vi "deploy alarm map.vi"() -> ()   [LabVIEW 2016, in "opSignIn.lvlib"]
uses:
  opSignIn.lvlib
  alarmMap.ctl
panel:
  in  "导入":bool
  in  "导出":bool
  in  "Project":i32(listbox)
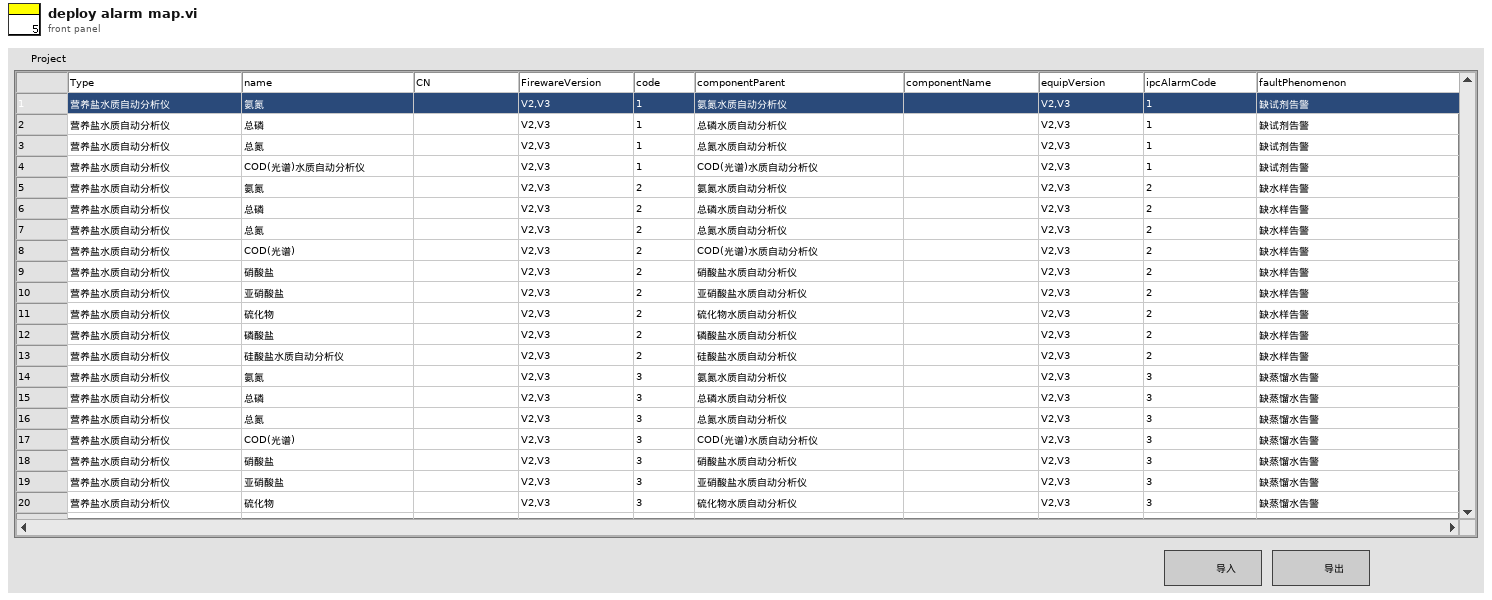
[diagram p1: front panel]
types:
  T1 = typedef "opSignIn.lvlib/alarmMap.ctl" = cluster{"name":string, "componentParentPath":string, "componentName":string, "equipVersion":string, "ipcAlarmCode":string, "faultName":string, "是否上报":string}
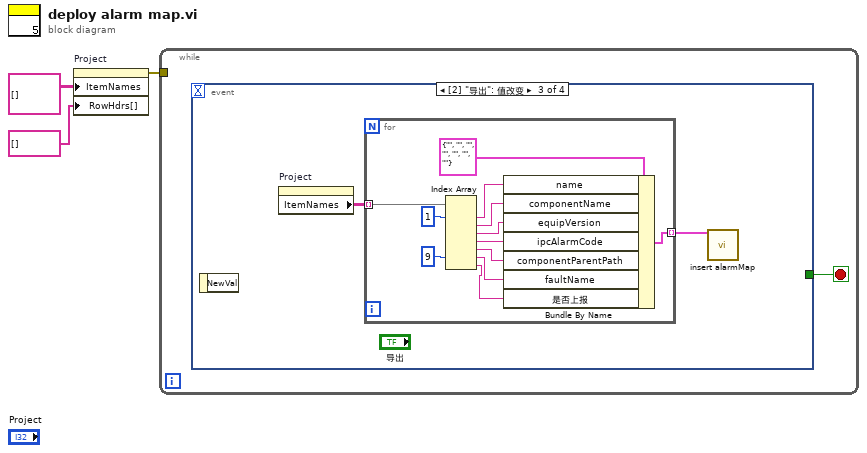
[diagram p0: block diagram]
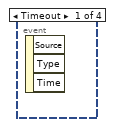
[diagram p2: hidden frame]
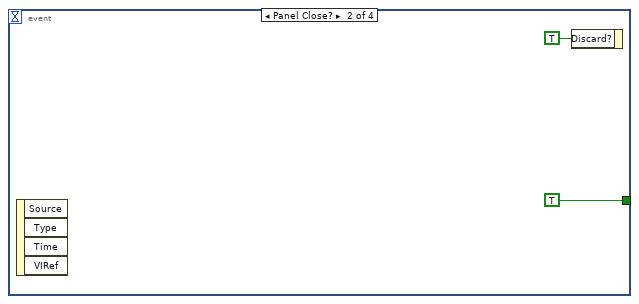
[diagram p3: hidden frame]
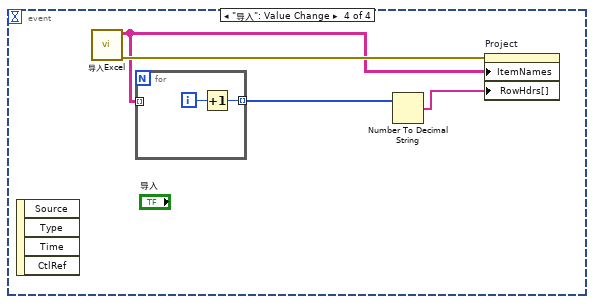
[diagram p4: hidden frame]
diagram:
  n1 = property on="Project" class="MCListbox (严格)"("ItemNames"=string[][] [] ("项名"), "RowHdrs[]"=string[] [] ("行首字符串[]")) -> (error out=w1:errorcluster)  [unwired: 2 in, 1 out]
  n2 = while {
    tunnel: w1 -> [_]
    stop <- w4 stop-if-true
    n3 = event shown="[2] \"导出\": 值改变" {
      selector: _ -> [_ _ _ _]
      dyn-events: _ -> [_ _ _ _]
      timeout: _ -> [_ _ _ _]
      tunnel: [_ TRUE _ _] -> w4
      event Timeout {
        n4 = event-data() -> ()  [unwired: 1 in, 3 out]
      }
      event Panel Close? {
        n5 = event-data() -> ()  [unwired: 1 in, 4 out]
        n6 = event-data("Discard?"=TRUE ("放弃？")) -> ()  [unwired: 1 in, 1 out]
      }
      event "导出": Value Change {
        n7 = event-data() -> ()  [unwired: 1 in, 1 out]
        n8 = property on="Project" class="MCListbox (严格)"() -> ("ItemNames"=w8:string[][])  [unwired: 2 in, 2 out]
        n9 = for {
          tunnel: w8 -> [w20] mode=indexing
          tunnel: [w13] -> w7 mode=indexing
          n10 = Index Array(array=w20, index #1=1 ("索引"), index #6=9 ("索引")) -> (element #1=w11:string, element #2=w18:string, element #3=w17:string, element #4=w16:string, element #5=w15:string, element #6=w14:string, element #7=w9:string)  [unwired: 5 in]
          n11 = Bundle By Name(cluster=T1 {"name"="", "componentParentPath"="", "componentName"="", "equipVersion"="", "ipcAlarmCode"="", "faultName"="", "是否上报"=""} ("alarmMap"), "name"=w11, "componentName"=w18, "equipVersion"=w17, "ipcAlarmCode"=w16, "componentParentPath"=w15, "faultName"=w14, "是否上报"=w9) -> (w13:T1)
        }
        n12 = call "insert alarmMap.vi"("alarmMap"=w7) -> ()  [unwired: 18 in, 1 out]
      }
      event "导入": Value Change {
        n13 = event-data() -> ()  [unwired: 1 in, 4 out]
        n14 = call "导入Excel.vi"() -> ("error out"=w24:errorcluster, "data"=w23:string[][])  [unwired: 10 in]
        n15 = for {
          tunnel: w23 -> [_] mode=indexing
          tunnel: [w25] -> w22 mode=indexing
          i -> [w26]
          n16 = Increment(x=w26) -> (x+1=w25:i32)
        }
        n17 = Number To Decimal String(number=w22) -> (decimal integer string=w21:string[])  [unwired: 1 in]
        n18 = property on="Project" class="MCListbox (严格)"(error in=w24, "ItemNames"=w23, "RowHdrs[]"=w21) -> ()  [unwired: 1 in, 2 out]
      }
    }
  }
